vi "Get Active Ctl Data.vi"(8 "error in":errorcluster, 11 "AC Comm in":refnum<class "AlicatCommBank.lvclass">) -> (0 "error out":errorcluster, 2 "DataOut":refnum<class "Data.lvclass">, 3 "AC Comm out":refnum<class "AlicatCommBank.lvclass">)   [LabVIEW 2013, in "Alicat.lvlib" / "AlicatCommBank.lvclass"]
uses:
  AlicatCommBank.lvclass
  Reusable/Data/Data.lvclass
  AlicatCommBank.lvclass/AlicatCommBank.ctl
  Alicat.lvclass
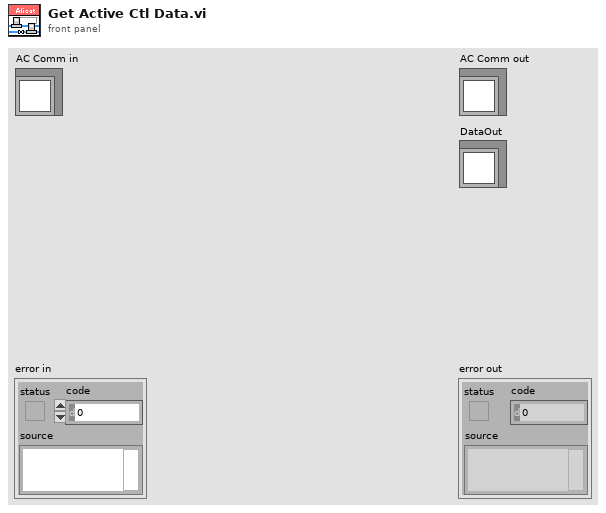
[diagram p1: front panel]
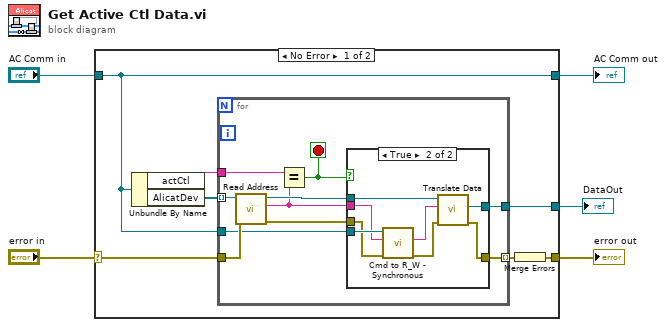
[diagram p0: block diagram]
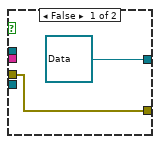
[diagram p2: hidden frame]
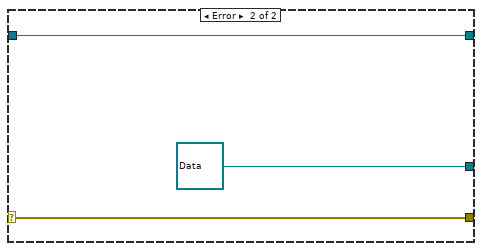
[diagram p3: hidden frame]
diagram:
  n1 = case shown="No Error" "error in" {
    selector: "error in" -> [w10 w35]
    tunnel: [w6 w35] -> w4
    tunnel: [w9 w34] -> w2
    tunnel: "AC Comm in" -> [w9 w34]
    tunnel: [w8 refnum<class "Data.lvclass"> refnum ("DataOut")] -> w1
    frame No Error {
      n2 = Unbundle By Name(w9) -> ("actCtl"=w11:string, "AlicatDev"=w12:refnum<class "Alicat.lvclass">[])
      n3 = for {
        tunnel: [w22] -> w7 mode=indexing
        tunnel: w10 -> [w21]
        tunnel: w12 -> [w19] mode=indexing
        tunnel: w11 -> [w17]
        tunnel: w9 -> [w15]
        tunnel: [w13] -> w8
        stop <- w16 stop-if-true
        n4 = call "Read Address.vi"("error in"=w21, "Alicat in"=w19) -> ("error out"=w20:errorcluster, "Address"=w14:string, "Alicat out"=w18:refnum<class "Alicat.lvclass">)  [unwired: 7 in]
        n5 = Equal?(x=w17, y=w14) -> (x = y?=w16:bool)
        n6 = case shown="True" w16 {
          tunnel: [w24 w27] -> w22
          tunnel: w20 -> [w24 w25]
          tunnel: w18 -> [_ w30]
          tunnel: w15 -> [_ w29]
          tunnel: w14 -> [_ w28]
          tunnel: [refnum<class "Data.lvclass"> refnum ("DataOut") w26] -> w13
          frame False {
          }
          frame True {
            n7 = call-dynamic "Cmd to R_W - Synchronous.vi"("error in"=w25, "write buffer"=w28, "Serial IO in"=w29) -> ("error out"=w31:errorcluster, "read buffer"=w32:string)  [unwired: 6 in, 1 out]
            n8 = call-dynamic "Translate Data.vi"("error in (no error)"=w31, "BufferIn"=w32, "Alicat in"=w30) -> ("error out"=w27:errorcluster, "DataOut"=w26:refnum<class "Data.lvclass">)  [unwired: 6 in, 1 out]
          }
        }
      }
      n9 = Merge Errors(w7) -> (w6:errorcluster)
    }
    frame Error {
    }
  }
  "error out" <- w4
  "AC Comm out" <- w2
  "DataOut" <- w1
